vi "no_IPE.vi"(8 "error in (no error)":errorcluster, 10 "data bus in":T1, 11 "Test Data in":T2) -> (0 "error out":errorcluster, 2 "data bus out":T1, 3 "Test Data out":T2)   [LabVIEW 2024, in "IPE Optimization Tester.lvlib"]
uses:
  IPE Optimization Tester.lvlib
  test_data--cluster.ctl
  SubVIs/data_bus--cluster.ctl
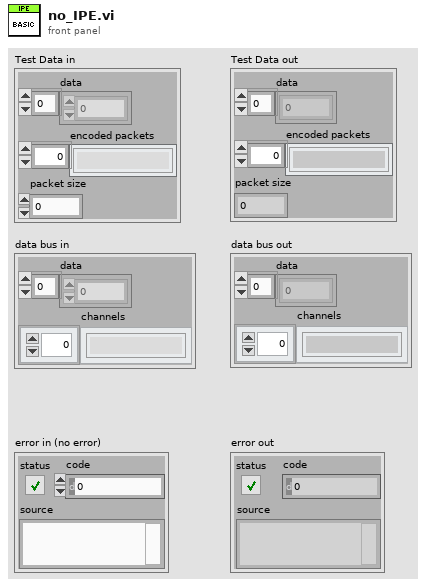
[diagram p1: front panel]
types:
  T1 = typedef "IPE Optimization Tester.lvlib/data_bus--cluster.ctl" = cluster{"data":dbl[], "channels":string[]}
  T2 = typedef "IPE Optimization Tester.lvlib/test_data--cluster.ctl" = cluster{"data":dbl[], "encoded packets":string[], "packet size":i32}
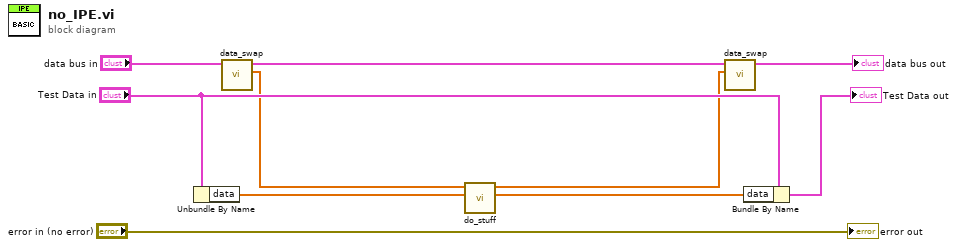
[diagram p0: block diagram]
diagram:
  n1 = Unbundle By Name("Test Data in") -> ("data"=w4:dbl[])
  n2 = call "data_swap.vi"("data bus in"="data bus in") -> ("data out"=w5:dbl[], "data bus out"=w6:T1)  [unwired: 9 in]
  n3 = call "do_stuff.vi"("live data in"=w4, "data bus in"=w5) -> ("live data out"=w2:dbl[], "data bus out"=w3:dbl[])  [unwired: 8 in]
  n4 = call "data_swap.vi"("data in"=w3, "data bus in"=w6) -> ("data bus out"=→"data bus out":T1)  [unwired: 8 in, 1 out]
  n5 = Bundle By Name(cluster="Test Data in", "data"=w2) -> (→"Test Data out":T2)
  "error out" <- "error in (no error)"
